vi "CreateSocket.vi"(8 "error in":errorcluster, 10 "Socket Type":T1=enum."REQ", 11 "context in":refnum<class "Context.lvclass">) -> (0 "error out":errorcluster, 2 "socket out":refnum<class "Socket.lvclass">, 3 "context out":refnum<class "Context.lvclass">)   [LabVIEW 2025, in "ZeroMQ.lvlib" / "Context.lvclass"]
doc: "Create a socket of flavour <b>socket type</b> in context <b>ctx in</b> and linger time <b>linger</b> milliseconds (time permitted after zmq_term to finish queued operations).\n\nNote that ZeroMQ creates sockets with infinite linger (ZMQ_LINGER) by default, which is undesirable in a managed environment like LabVIEW since it hangs the parent process. But set it to -1 should infinite linger be required.\n\nDetailed API documentation: http://api.zeromq.org/3-2:zmq-socket"
uses:
  Context.lvclass
  libzmq-v143-mt-4_3_6/ctls/SocketType.ctl
  Socket.lvclass
  Context.lvclass/Context.ctl
  libzmq-v143-mt-4_3_6/LibZMQ.lvlib
panel:
  # "ØMQ"
  # "labview"
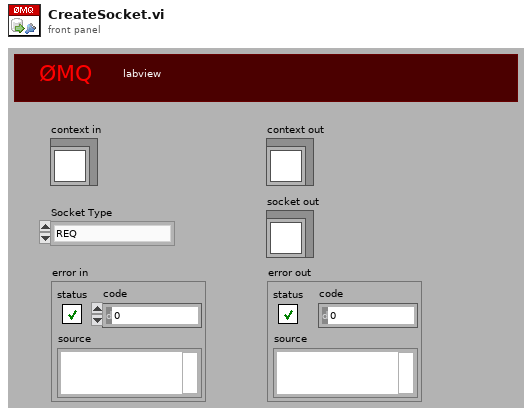
[diagram p1: front panel]
types:
  T1 = typedef "LibZMQ.lvlib/SocketType.ctl" = enum8{"PAIR", "PUB", "SUB", "REQ", "REP", "DEALER", "ROUTER", "PULL", "PUSH", "XPUB", "XSUB", "STREAM"}
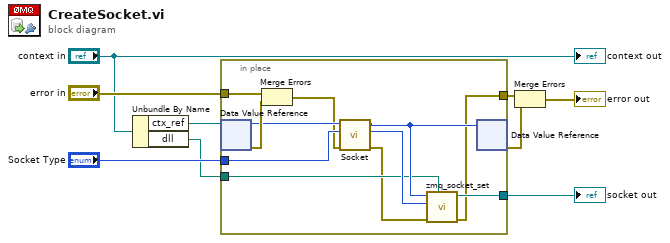
[diagram p0: block diagram]
diagram:
  n1 = Unbundle By Name("context in") -> ("ctx_ref"=w4:refnum<data-value>, "dll"=w1:path)
  n2 = in-place {
    in-place-border: "error in" -> [w20]
    in-place-border: "Socket Type" -> [w15]
    in-place-border: [w10] -> w6
    in-place-border: [w19] -> w5
    in-place-border: w1 -> [w12]
    n3 = in-place-dvr #1(w4) -> (w17:u64, w18:errorcluster)
    n4 = Merge Errors(w20, w18) -> (w13:errorcluster)
    n5 = call "Socket.vi"("error in (no error)"=w13, "Socket Type"=w15, "ctx in"=w17) -> ("error out"=w11:errorcluster, "s_"=w14:u64, "ctx out"=w16:u64)  [unwired: 6 in]
    n6 = call "zmq_socket_set.vi"("dll"=w12, "error in"=w11, "socket"=w14, "context"=w16) -> ("error out"=w10:errorcluster, "socket out"=w19:refnum<class "Socket.lvclass">)  [unwired: 6 in]
    n7 = in-place-dvr #1(w16) -> (w2:errorcluster)  [unwired: 1 out]
  }
  "socket out" <- w5
  n8 = Merge Errors(w6, w2) -> (→"error out":errorcluster)
  "context out" <- "context in"
